vi "Terminate Sequence.vi"(4 "Buffers":T1, 6 "Terminal Options":T2={"Implied CR with LF"=TRUE, "Local Echo"=FALSE, "Tab Width"=8, "Color Scheme"={"Black"=2302755, "Red"=16711695, "Green"=9232651, "Yellow"=16759040, "Blue"=36344, "Magenta"=7160742, "Cyan"=55531, "White"=15132390, "Bright Black"=4473924, "Bright Red"=16721728, "Bright Green"=11264347, "Bright Yellow"=16765506, "Bright Blue"=37631, "Bright Magenta"=10117099, "Bright Cyan"=6815728, "Bright White"=16777215}, "Default FG"=37, "Default BG"=90, "History Length"=5000, "Font Face"="Fixedsys", "Font Size"=14, "Rows"=24, "Cols"=80} {"Default BG" items=["Black"=30, "Red"=31, "Green"=32, "Yellow"=33, "Blue"=34, "Magenta"=35, "Cyan"=36, "White"=37, "Gray"=90, "Bright Red"=91, "Bright Green"=92, "Bright Yellow"=93, "Bright Blue"=94, "Bright Magenta"=95, "Bright Cyan"=96, "Bright White"=97]; "Default FG" items=["Black"=30, "Red"=31, "Green"=32, "Yellow"=33, "Blue"=34, "Magenta"=35, "Cyan"=36, "White"=37, "Gray"=90, "Bright Red"=91, "Bright Green"=92, "Bright Yellow"=93, "Bright Blue"=94, "Bright Magenta"=95, "Bright Cyan"=96, "Bright White"=97]}, 10 "Terminator":u8, 11 "Parse State In":T5) -> (3 "Parse State":T5)   [LabVIEW 2020, in "Terminal.lvlib" / "Terminal.lvclass"]
uses:
  Terminal.lvclass
  Terminal.lvclass/Terminal.ctl
  Color.ctl
  Terminal.lvlib
  TermBuffer/TermBuffer.lvclass
  Buffer.ctl
  Parse State.ctl
  Color Scheme.ctl
  Terminal Options.ctl
  Buffers.ctl
  Position.ctl
  Cursor.ctl
  Text Attributes.ctl
  Buffer State.ctl
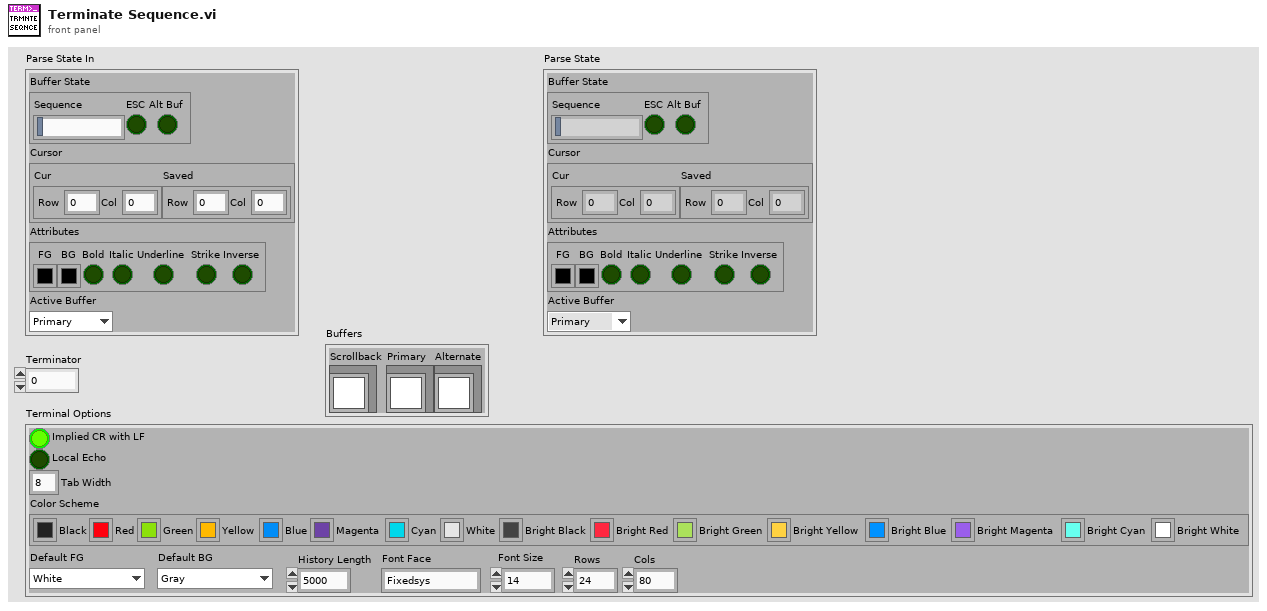
[diagram p1: front panel]
types:
  T1 = typedef "Terminal.lvlib/Terminal.lvclass/Buffers.ctl" = cluster{"Scrollback":refnum<class "TermBuffer.lvclass">, "Primary":refnum<class "TermBuffer.lvclass">, "Alternate":refnum<class "TermBuffer.lvclass">}
  T2 = typedef "Terminal.lvlib/Terminal Options.ctl" = cluster{"Implied CR with LF":bool, "Local Echo":bool, "Tab Width":i32, "Color Scheme":T3, "Default FG":T4, "Default BG":T4, "History Length":i32, "Font Face":string, "Font Size":i16, "Rows":i32, "Cols":i32}
  T3 = typedef "Terminal.lvlib/Color Scheme.ctl" = cluster{"Black":u32, "Red":u32, "Green":u32, "Yellow":u32, "Blue":u32, "Magenta":u32, "Cyan":u32, "White":u32, "Bright Black":u32, "Bright Red":u32, "Bright Green":u32, "Bright Yellow":u32, "Bright Blue":u32, "Bright Magenta":u32, "Bright Cyan":u32, "Bright White":u32}
  T4 = typedef "Terminal.lvlib/Color.ctl" = i8
  T5 = typedef "Terminal.lvlib/Terminal.lvclass/Parse State.ctl" = cluster{"Buffer State":T6, "Cursor":T7, "Attributes":T9, "Active Buffer":T10}
  T6 = typedef "Terminal.lvlib/Terminal.lvclass/Buffer State.ctl" = cluster{"Sequence":string, "ESC":bool, "Alt Buf":bool}
  T7 = typedef "Terminal.lvlib/Terminal.lvclass/Cursor.ctl" = cluster{"Cur":T8, "Saved":T8}
  T8 = typedef "Terminal.lvlib/Terminal.lvclass/Position.ctl" = cluster{"Row":i32, "Col":i32}
  T9 = typedef "Terminal.lvlib/Text Attributes.ctl" = cluster{"FG":u32, "BG":u32, "Bold":bool, "Italic":bool, "Underline":bool, "Strike":bool, "Inverse":bool}
  T10 = typedef "Terminal.lvlib/Buffer.ctl" = enum16{"Primary", "Alternate"}
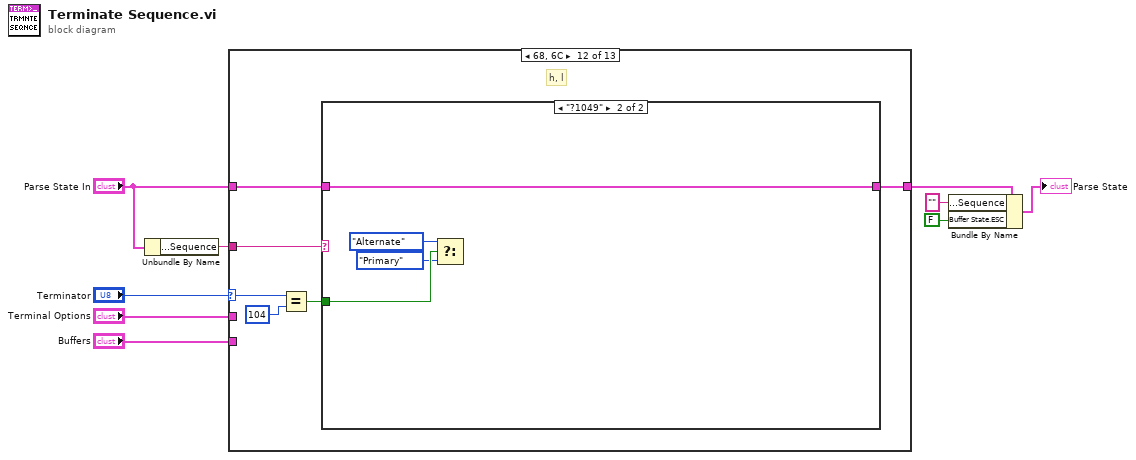
[diagram p0: block diagram]
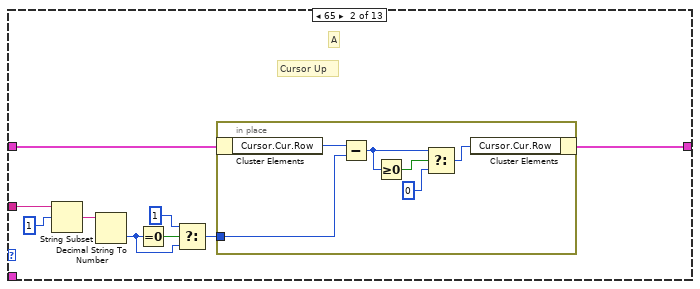
[diagram p3: hidden frame]
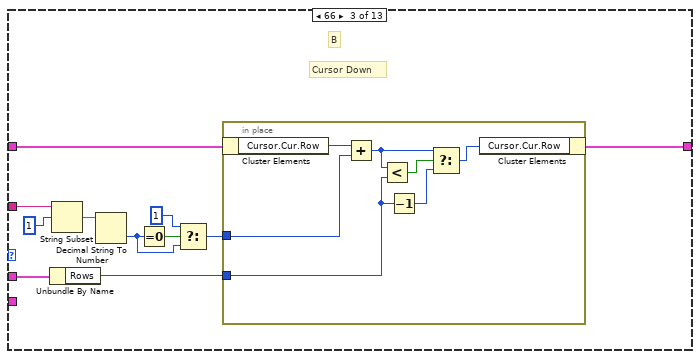
[diagram p4: hidden frame]
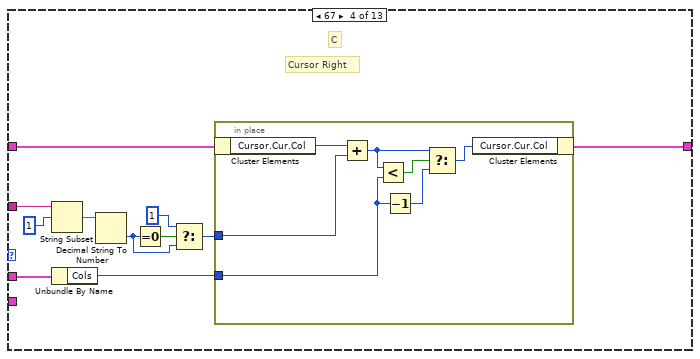
[diagram p5: hidden frame]
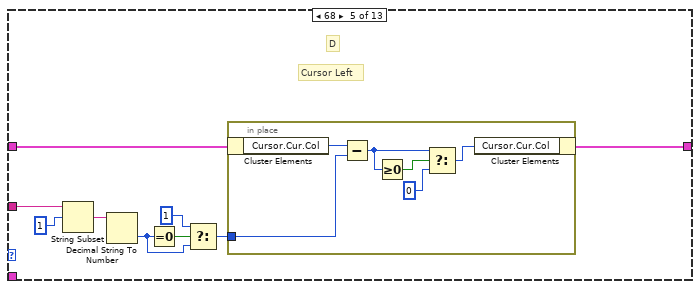
[diagram p6: hidden frame]
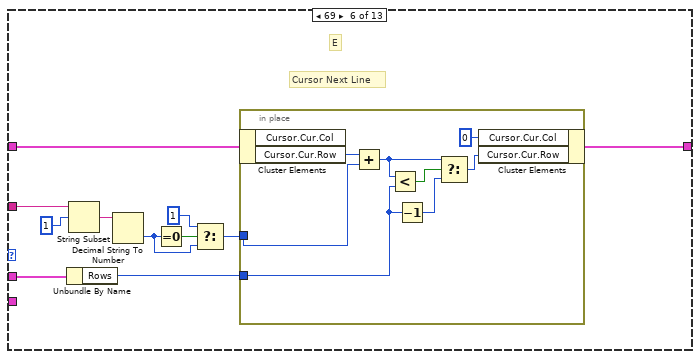
[diagram p7: hidden frame]
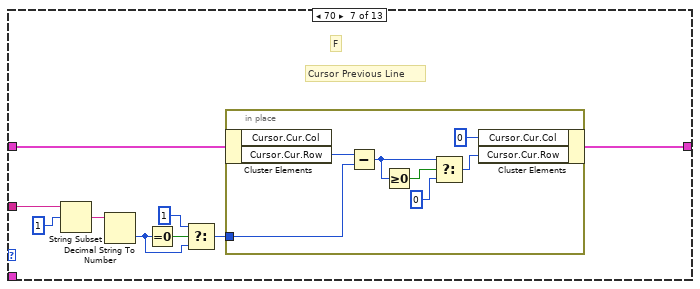
[diagram p8: hidden frame]
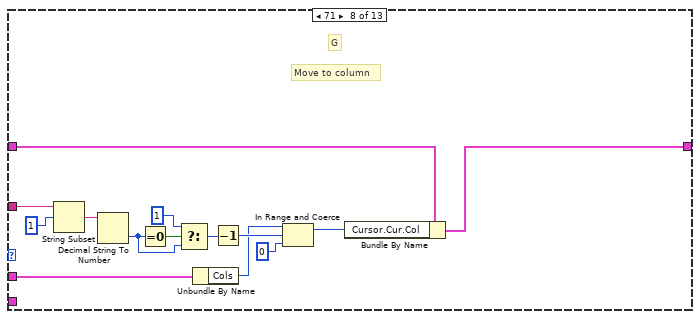
[diagram p9: hidden frame]
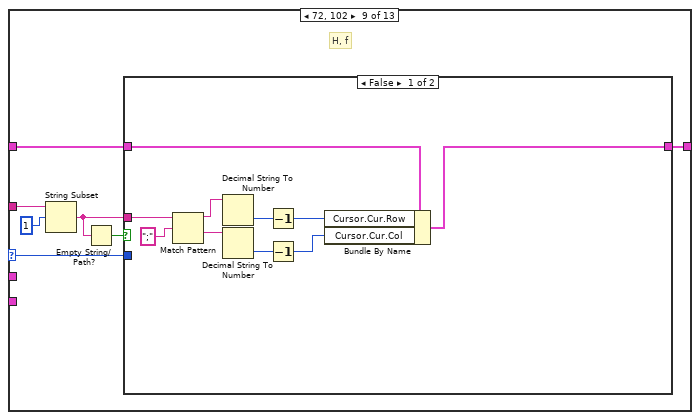
[diagram p10: hidden frame]
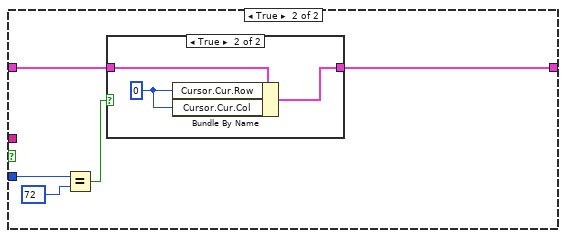
[diagram p11: hidden frame]
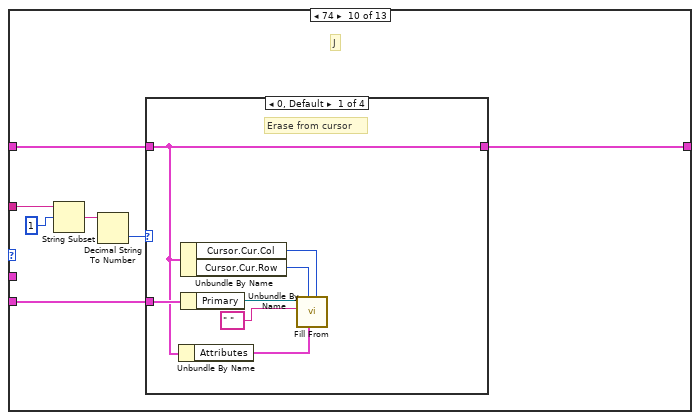
[diagram p13: hidden frame]
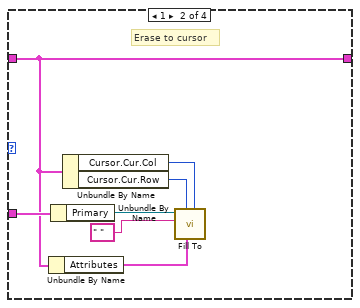
[diagram p14: hidden frame]
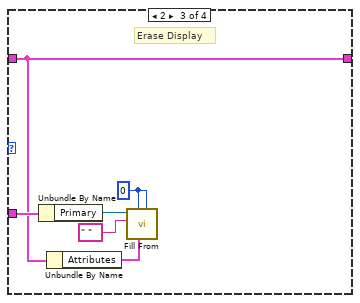
[diagram p15: hidden frame]
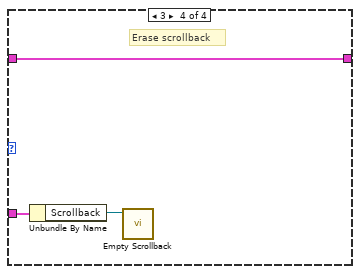
[diagram p16: hidden frame]
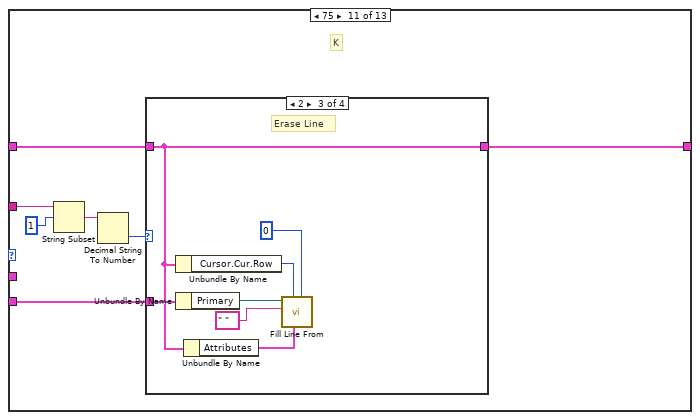
[diagram p17: hidden frame]
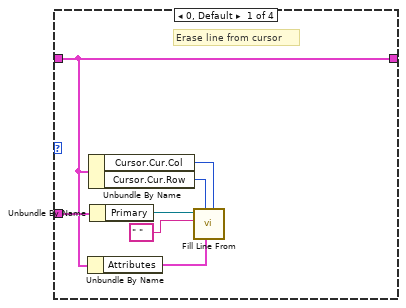
[diagram p18: hidden frame]
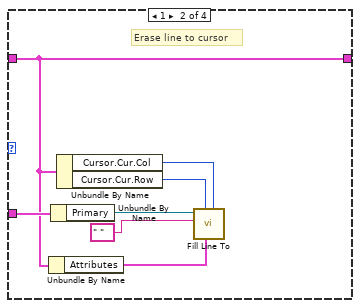
[diagram p19: hidden frame]
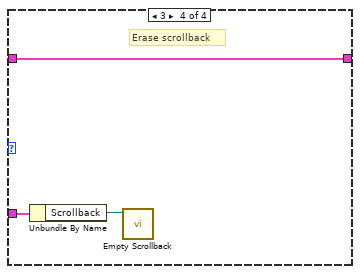
[diagram p20: hidden frame]
diagram:
  n1 = Unbundle By Name("Parse State In") -> ("Buffer State.Sequence"=w7:string)
  n2 = case shown="68, 6C" "Terminator" {
    selector: "Terminator" -> [_ _ _ _ _ _ _ _ w126 _ _ w216 _]
    tunnel: "Parse State In" -> [w10 w16 w33 w51 w63 w80 w97 w114 w130 w155 w185 w218 w226]
    tunnel: w7 -> [_ w19 w36 w54 w64 w79 w98 w120 w132 w156 w186 w214 w229]
    tunnel: [w10 w15 w32 w50 w62 w77 w96 w112 w128 w152 w182 w217 w225] -> w6
    tunnel: "Terminal Options" -> [_ _ w31 w49 _ w78 _ w116 _ _ _ _ w224]
    tunnel: "Buffers" -> [_ _ _ _ _ _ _ _ _ w153 w183 _ _]
    frame Default {
    }
    frame 65 {
      # "Cursor Up"
      # "A"
      n3 = String Subset(string=w19, offset (0)=1) -> (substring=w17:string)  [unwired: 1 in]
      n4 = Decimal String To Number(string=w17) -> (number=w12:i32)  [unwired: 2 in, 1 out]
      n5 = Equal To 0?(x=w12) -> (x = 0?=w14:bool)
      n6 = Select(t=1, s=w14, f=w12) -> (s? t:f=w11:i32)
      n7 = in-place {
        in-place-border: w11 -> [w24]
        n8 = in-place-cluster #1(w16) -> ("Cursor.Cur.Row"=w25:i32)
        n9 = Subtract(x=w25, y=w24) -> (x-y=w22:i32)
        n10 = Greater Or Equal To 0?(x=w22) -> (x >= 0?=w23:bool)
        n11 = Select(t=w22, s=w23, f=0) -> (s? t:f=w20:i32)
        n12 = in-place-cluster #1("Cursor.Cur.Row"=w20) -> (w15:T5)
      }
    }
    frame 66 {
      # "Cursor Down"
      # "B"
      n13 = Unbundle By Name(w31) -> ("Rows"=w30:i32)
      n14 = String Subset(string=w36, offset (0)=1) -> (substring=w34:string)  [unwired: 1 in]
      n15 = Decimal String To Number(string=w34) -> (number=w27:i32)  [unwired: 2 in, 1 out]
      n16 = Equal To 0?(x=w27) -> (x = 0?=w29:bool)
      n17 = Select(t=1, s=w29, f=w27) -> (s? t:f=w26:i32)
      n18 = in-place {
        in-place-border: w30 -> [w39]
        in-place-border: w26 -> [w37]
        n19 = in-place-cluster #2(w33) -> ("Cursor.Cur.Row"=w43:i32)
        n20 = Add(x=w43, y=w37) -> (x+y=w41:i32)
        n21 = Less?(x=w41, y=w39) -> (x < y?=w40:bool)
        n22 = Decrement(x=w39) -> (x-1=w38:i32)
        n23 = Select(t=w41, s=w40, f=w38) -> (s? t:f=w42:i32)
        n24 = in-place-cluster #2("Cursor.Cur.Row"=w42) -> (w32:T5)
      }
    }
    frame 67 {
      # "Cursor Right"
      # "C"
      n25 = String Subset(string=w54, offset (0)=1) -> (substring=w52:string)  [unwired: 1 in]
      n26 = Unbundle By Name(w49) -> ("Cols"=w48:i32)
      n27 = Decimal String To Number(string=w52) -> (number=w46:i32)  [unwired: 2 in, 1 out]
      n28 = Equal To 0?(x=w46) -> (x = 0?=w47:bool)
      n29 = Select(t=1, s=w47, f=w46) -> (s? t:f=w44:i32)
      n30 = in-place {
        in-place-border: w44 -> [w60]
        in-place-border: w48 -> [w56]
        n31 = in-place-cluster #3(w51) -> ("Cursor.Cur.Col"=w61:i32)
        n32 = Add(x=w61, y=w60) -> (x+y=w58:i32)
        n33 = Less?(x=w58, y=w56) -> (x < y?=w57:bool)
        n34 = Decrement(x=w56) -> (x-1=w55:i32)
        n35 = Select(t=w58, s=w57, f=w55) -> (s? t:f=w59:i32)
        n36 = in-place-cluster #3("Cursor.Cur.Col"=w59) -> (w50:T5)
      }
    }
    frame 68 {
      # "Cursor Left"
      # "D"
      n37 = String Subset(string=w64, offset (0)=1) -> (substring=w69:string)  [unwired: 1 in]
      n38 = Decimal String To Number(string=w69) -> (number=w66:i32)  [unwired: 2 in, 1 out]
      n39 = Equal To 0?(x=w66) -> (x = 0?=w68:bool)
      n40 = Select(t=1, s=w68, f=w66) -> (s? t:f=w65:i32)
      n41 = in-place {
        in-place-border: w65 -> [w75]
        n42 = in-place-cluster #4(w63) -> ("Cursor.Cur.Col"=w76:i32)
        n43 = Subtract(x=w76, y=w75) -> (x-y=w73:i32)
        n44 = Greater Or Equal To 0?(x=w73) -> (x >= 0?=w74:bool)
        n45 = Select(t=w73, s=w74, f=0) -> (s? t:f=w71:i32)
        n46 = in-place-cluster #4("Cursor.Cur.Col"=w71) -> (w62:T5)
      }
    }
    frame 69 {
      # "Cursor Next Line"
      # "E"
      n47 = Unbundle By Name(w78) -> ("Rows"=w85:i32)
      n48 = String Subset(string=w79, offset (0)=1) -> (substring=w86:string)  [unwired: 1 in]
      n49 = Decimal String To Number(string=w86) -> (number=w82:i32)  [unwired: 2 in, 1 out]
      n50 = Equal To 0?(x=w82) -> (x = 0?=w84:bool)
      n51 = Select(t=1, s=w84, f=w82) -> (s? t:f=w81:i32)
      n52 = in-place {
        in-place-border: w85 -> [w91]
        in-place-border: w81 -> [w89]
        n53 = in-place-cluster #5(w80) -> ("Cursor.Cur.Row"=w95:i32)  [unwired: 1 out]
        n54 = Add(x=w95, y=w89) -> (x+y=w93:i32)
        n55 = Less?(x=w93, y=w91) -> (x < y?=w92:bool)
        n56 = Decrement(x=w91) -> (x-1=w90:i32)
        n57 = Select(t=w93, s=w92, f=w90) -> (s? t:f=w94:i32)
        n58 = in-place-cluster #5("Cursor.Cur.Col"=0 ("Cur Col"), "Cursor.Cur.Row"=w94) -> (w77:T5)
      }
    }
    frame 70 {
      # "Cursor Previous Line"
      # "F"
      n59 = String Subset(string=w98, offset (0)=1) -> (substring=w103:string)  [unwired: 1 in]
      n60 = Decimal String To Number(string=w103) -> (number=w100:i32)  [unwired: 2 in, 1 out]
      n61 = Equal To 0?(x=w100) -> (x = 0?=w102:bool)
      n62 = Select(t=1, s=w102, f=w100) -> (s? t:f=w99:i32)
      n63 = in-place {
        in-place-border: w99 -> [w110]
        n64 = in-place-cluster #6(w97) -> ("Cursor.Cur.Row"=w111:i32)  [unwired: 1 out]
        n65 = Subtract(x=w111, y=w110) -> (x-y=w108:i32)
        n66 = Greater Or Equal To 0?(x=w108) -> (x >= 0?=w109:bool)
        n67 = Select(t=w108, s=w109, f=0) -> (s? t:f=w106:i32)
        n68 = in-place-cluster #6("Cursor.Cur.Col"=0 ("Cur Col"), "Cursor.Cur.Row"=w106) -> (w96:T5)
      }
    }
    frame 71 {
      # "Move to column"
      # "G"
      n69 = String Subset(string=w120, offset (0)=1) -> (substring=w124:string)  [unwired: 1 in]
      n70 = Decimal String To Number(string=w124) -> (number=w121:i32)  [unwired: 2 in, 1 out]
      n71 = Equal To 0?(x=w121) -> (x = 0?=w123:bool)
      n72 = Select(t=1, s=w123, f=w121) -> (s? t:f=w119:i32)
      n73 = Unbundle By Name(w116) -> ("Cols"=w115:i32)
      n74 = Decrement(x=w119) -> (x-1=w118:i32)
      n75 = In Range and Coerce(upper limit=w115, x=w118, lower limit=0) -> (coerced(x)=w113:i32)  [unwired: 1 out]
      n76 = Bundle By Name(cluster=w114, "Cursor.Cur.Col"=w113) -> (w112:T5)
    }
    frame 72, 102 {
      # "H, f"
      n77 = String Subset(string=w132, offset (0)=1) -> (substring=w127:string)  [unwired: 1 in]
      n78 = Empty String/Path?(string/path=w127) -> (empty?=w129:bool)
      n79 = case shown="False" w129 {
        tunnel: w130 -> [w138 w147]
        tunnel: [w135 w146] -> w128
        tunnel: w127 -> [w142 _]
        tunnel: w126 -> [_ w145]
        frame False {
          n80 = Match Pattern(string=w142, regular expression=";") -> (before substring=w139:string, after substring=w140:string)  [unwired: 1 in, 2 out]
          n81 = Decimal String To Number(string=w139) -> (number=w137:i32)  [unwired: 2 in, 1 out]
          n82 = Decimal String To Number(string=w140) -> (number=w136:i32)  [unwired: 2 in, 1 out]
          n83 = Decrement(x=w137) -> (x-1=w134:i32)
          n84 = Decrement(x=w136) -> (x-1=w133:i32)
          n85 = Bundle By Name(cluster=w138, "Cursor.Cur.Row"=w134, "Cursor.Cur.Col"=w133) -> (w135:T5)
        }
        frame True {
          n86 = Equal?(x=w145, y=u8 72) -> (x = y?=w143:bool)
          n87 = case shown="True" w143 {
            tunnel: w147 -> [w148 w151]
            tunnel: [w148 w149] -> w146
            frame False {
            }
            frame True {
              w150 = 0 ("Cur Row")
              n88 = Bundle By Name(cluster=w151, "Cursor.Cur.Row"=w150, "Cursor.Cur.Col"=w150) -> (w149:T5)
            }
          }
        }
      }
    }
    frame 74 {
      # "J"
      n89 = String Subset(string=w156, offset (0)=1) -> (substring=w157:string)  [unwired: 1 in]
      n90 = Decimal String To Number(string=w157) -> (number=w154:i32)  [unwired: 2 in, 1 out]
      n91 = case shown="0, Default" w154 {
        tunnel: w155 -> [w161 w166 w174 w181]
        tunnel: w153 -> [w165 w167 w178 w180]
        tunnel: [w161 w166 w174 w181] -> w152
        frame 0, Default {
          # "Erase from cursor"
          n92 = Unbundle By Name(w161) -> ("Attributes"=w159:T9)
          n93 = Unbundle By Name(w161) -> ("Cursor.Cur.Col"=w162:i32, "Cursor.Cur.Row"=w163:i32)
          n94 = Unbundle By Name(w165) -> ("Primary"=w164:refnum<class "TermBuffer.lvclass">)
          n95 = call "Fill From.vi"("Col"=w162, "Attributes"=w159, "Row"=w163, "Char"=" ", "TermBuffer in"=w164) -> ()  [unwired: 5 in, 2 out]
        }
        frame 1 {
          # "Erase to cursor"
          n96 = Unbundle By Name(w166) -> ("Attributes"=w168:T9)
          n97 = Unbundle By Name(w167) -> ("Primary"=w172:refnum<class "TermBuffer.lvclass">)
          n98 = Unbundle By Name(w166) -> ("Cursor.Cur.Col"=w170:i32, "Cursor.Cur.Row"=w171:i32)
          n99 = call "Fill To.vi"("Col"=w170, "Attributes"=w168, "Row"=w171, "Char"=" ", "TermBuffer in"=w172) -> ()  [unwired: 5 in, 2 out]
        }
        frame 2 {
          w175 = 0 ("Row")
          # "Erase Display"
          n100 = Unbundle By Name(w178) -> ("Primary"=w177:refnum<class "TermBuffer.lvclass">)
          n101 = Unbundle By Name(w174) -> ("Attributes"=w173:T9)
          n102 = call "Fill From.vi"("Col"=w175, "Attributes"=w173, "Row"=w175, "Char"=" ", "TermBuffer in"=w177) -> ()  [unwired: 5 in, 2 out]
        }
        frame 3 {
          # "Erase scrollback"
          n103 = Unbundle By Name(w180) -> ("Scrollback"=w179:refnum<class "TermBuffer.lvclass">)
          n104 = call "Empty Scrollback.vi"("TermBuffer in"=w179) -> ()  [unwired: 9 in, 2 out]
        }
      }
    }
    frame 75 {
      # "K"
      n105 = String Subset(string=w186, offset (0)=1) -> (substring=w187:string)  [unwired: 1 in]
      n106 = Decimal String To Number(string=w187) -> (number=w184:i32)  [unwired: 2 in, 1 out]
      n107 = case shown="2" w184 {
        tunnel: w185 -> [w191 w196 w206 w212]
        tunnel: w183 -> [w195 w197 w209 w211]
        tunnel: [w191 w196 w206 w212] -> w182
        frame 0, Default {
          # "Erase line from cursor"
          n108 = Unbundle By Name(w191) -> ("Attributes"=w189:T9)
          n109 = Unbundle By Name(w191) -> ("Cursor.Cur.Col"=w192:i32, "Cursor.Cur.Row"=w193:i32)
          n110 = Unbundle By Name(w195) -> ("Primary"=w194:refnum<class "TermBuffer.lvclass">)
          n111 = call "Fill Line From.vi"("Col"=w192, "Attributes"=w189, "Row"=w193, "Char"=" ", "TermBuffer in"=w194) -> ()  [unwired: 5 in, 2 out]
        }
        frame 1 {
          # "Erase line to cursor"
          n112 = Unbundle By Name(w196) -> ("Attributes"=w198:T9)
          n113 = Unbundle By Name(w197) -> ("Primary"=w202:refnum<class "TermBuffer.lvclass">)
          n114 = Unbundle By Name(w196) -> ("Cursor.Cur.Col"=w200:i32, "Cursor.Cur.Row"=w201:i32)
          n115 = call "Fill Line To.vi"("Col"=w200, "Attributes"=w198, "Row"=w201, "Char"=" ", "TermBuffer in"=w202) -> ()  [unwired: 5 in, 2 out]
        }
        frame 2 {
          # "Erase Line"
          n116 = Unbundle By Name(w206) -> ("Cursor.Cur.Row"=w205:i32)
          n117 = Unbundle By Name(w209) -> ("Primary"=w208:refnum<class "TermBuffer.lvclass">)
          n118 = Unbundle By Name(w206) -> ("Attributes"=w203:T9)
          n119 = call "Fill Line From.vi"("Col"=0, "Attributes"=w203, "Row"=w205, "Char"=" ", "TermBuffer in"=w208) -> ()  [unwired: 5 in, 2 out]
        }
        frame 3 {
          # "Erase scrollback"
          n120 = Unbundle By Name(w211) -> ("Scrollback"=w210:refnum<class "TermBuffer.lvclass">)
          n121 = call "Empty Scrollback.vi"("TermBuffer in"=w210) -> ()  [unwired: 9 in, 2 out]
        }
      }
    }
    frame 104, 108 {
      # "h, l"
      n122 = Equal?(x=w216, y=u8 104) -> (x = y?=w213:bool)
      n123 = case shown="\"?1049\"" w214 {
        tunnel: w218 -> [w219 w220]
        tunnel: [w219 w220] -> w217
        tunnel: w213 -> [_ w223]
        frame Default {
        }
        frame "?1049" {
          n124 = Select(t=Buffer."Alternate" ("Buffer"), s=w223, f=Buffer."Primary" ("Buffer")) -> ()  [unwired: 1 out]
        }
      }
    }
    frame 109 {
      w230 = 1 ("length (rest)")
      # "Character mode / color"
      # "m"
      n125 = String Subset(string=w229, offset (0)=w230) -> (substring=w228:string)  [unwired: 1 in]
      n126 = String Subset(string=w229, length (rest)=w230) -> (substring=w232:string)  [unwired: 1 in]
      n127 = Equal?(x=w232, y="[") -> (x = y?=w227:bool)
      n128 = case shown="True" w227 {
        tunnel: w228 -> [_ w239]
        tunnel: w226 -> [w233 w236]
        tunnel: [w233 w235] -> w225
        tunnel: w224 -> [_ w234]
        frame False {
        }
        frame True {
          n129 = call <vilib>:"Delimited String to 1D String Array.vi"("delimiter"=";", "delimited string"=w239) -> ("string array"=w237:string[])  [unwired: 9 in]
          n130 = for {
            tunnel: w237 -> [w242] mode=indexing
            shift-right: [w241] -> w235
            shift-left: w236 -> [w243]
            tunnel: w234 -> [w240]
            n131 = case shown="\"0\"" w242 {
              tunnel: w243 -> [w244 w253 w256 w257 w260 w263 w264 w267 w268 w271 w274 w277 w280 w281 w284 w285 w288 w291 w297 w303 w309 w315 w321 w327 w333 w340 w345 w351 w357 w363 w369 w375 w381 w387 w394 w399 w405 w411 w417 w423 w429 w435 w441 w447 w453 w459 w465 w471 w477 w483 w489]
              tunnel: [w244 w251 w254 w257 w258 w261 w264 w265 w268 w269 w272 w276 w278 w281 w282 w285 w286 w289 w295 w301 w307 w313 w319 w325 w331 w338 w343 w349 w355 w361 w367 w373 w379 w385 w392 w397 w403 w409 w415 w421 w427 w433 w439 w445 w451 w457 w463 w469 w475 w481 w487] -> w241
              tunnel: w240 -> [_ w250 _ _ _ _ _ _ _ _ _ _ _ _ _ _ _ w294 w300 w306 w312 w318 w324 w330 w336 w342 w348 w354 w360 w366 w372 w378 w384 w390 w396 w402 w408 w414 w420 w426 w432 w438 w444 w450 w456 w462 w468 w474 w480 w486 w492]
              frame Default {
              }
              frame "0" {
                w252 = FALSE ("Bold")
                n132 = Unbundle By Name(w250) -> ("Color Scheme"=w247:T3, "Default FG"=w249:T4, "Default BG"=w248:T4)
                n133 = call "Select Color.vi"("Color"=w249, "Color Scheme"=w247) -> ("Color Value"=w246:u32)  [unwired: 9 in]
                n134 = call "Select Color.vi"("Color"=w248, "Color Scheme"=w247) -> ("Color Value"=w245:u32)  [unwired: 9 in]
                n135 = Bundle By Name(cluster=w253, "Attributes.Bold"=w252, "Attributes.Italic"=w252, "Attributes.Underline"=w252, "Attributes.Strike"=w252, "Attributes.Inverse"=w252, "Attributes.FG"=w246, "Attributes.BG"=w245) -> (w251:T5)
              }
              frame "1" {
                n136 = Bundle By Name(cluster=w256, "Attributes.Bold"=TRUE ("Bold")) -> (w254:T5)
              }
              frame "2" {
                # "Dim/Faint On"
              }
              frame "3" {
                n137 = Bundle By Name(cluster=w260, "Attributes.Italic"=TRUE ("Italic")) -> (w258:T5)
              }
              frame "4" {
                n138 = Bundle By Name(cluster=w263, "Attributes.Underline"=TRUE ("Underline")) -> (w261:T5)
              }
              frame "5" {
                # "#TODO\nBlink On"
              }
              frame "7" {
                n139 = Bundle By Name(cluster=w267, "Attributes.Inverse"=TRUE ("Inverse")) -> (w265:T5)
              }
              frame "8" {
                # "Invisible On"
              }
              frame "9" {
                n140 = Bundle By Name(cluster=w271, "Attributes.Strike"=TRUE ("Strike")) -> (w269:T5)
              }
              frame "22" {
                n141 = Bundle By Name(cluster=w274, "Attributes.Bold"=FALSE ("Bold")) -> (w272:T5)
              }
              frame "23" {
                n142 = Bundle By Name(cluster=w277, "Attributes.Italic"=FALSE ("Italic")) -> (w276:T5)
              }
              frame "24" {
                n143 = Bundle By Name(cluster=w280, "Attributes.Underline"=FALSE ("Underline")) -> (w278:T5)
              }
              frame "25" {
                # "#TODO\nBlink Off"
              }
              frame "27" {
                n144 = Bundle By Name(cluster=w284, "Attributes.Inverse"=FALSE ("Inverse")) -> (w282:T5)
              }
              frame "28" {
                # "Invisible Off"
              }
              frame "29" {
                n145 = Bundle By Name(cluster=w288, "Attributes.Strike"=FALSE ("Strike")) -> (w286:T5)
              }
              frame "30" {
                w292 = T4 30 items=["Black"=30, "Red"=31, "Green"=32, "Yellow"=33, "Blue"=34, "Magenta"=35, "Cyan"=36, "White"=37, "Gray"=90, "Bright Red"=91, "Bright Green"=92, "Bright Yellow"=93, "Bright Blue"=94, "Bright Magenta"=95, "Bright Cyan"=96, "Bright White"=97] ("Color")
                n146 = Unbundle By Name(w294) -> ("Color Scheme"=w293:T3)
                n147 = call "Select Color.vi"("Color"=w292, "Color Scheme"=w293) -> ("Color Value"=w290:u32)  [unwired: 9 in]
                n148 = Bundle By Name(cluster=w291, "Attributes.FG"=w290) -> (w289:T5)
              }
              frame "31" {
                w298 = T4 31 items=["Black"=30, "Red"=31, "Green"=32, "Yellow"=33, "Blue"=34, "Magenta"=35, "Cyan"=36, "White"=37, "Gray"=90, "Bright Red"=91, "Bright Green"=92, "Bright Yellow"=93, "Bright Blue"=94, "Bright Magenta"=95, "Bright Cyan"=96, "Bright White"=97] ("Color")
                n149 = Unbundle By Name(w300) -> ("Color Scheme"=w299:T3)
                n150 = call "Select Color.vi"("Color"=w298, "Color Scheme"=w299) -> ("Color Value"=w296:u32)  [unwired: 9 in]
                n151 = Bundle By Name(cluster=w297, "Attributes.FG"=w296) -> (w295:T5)
              }
              frame "32" {
                w304 = T4 32 items=["Black"=30, "Red"=31, "Green"=32, "Yellow"=33, "Blue"=34, "Magenta"=35, "Cyan"=36, "White"=37, "Gray"=90, "Bright Red"=91, "Bright Green"=92, "Bright Yellow"=93, "Bright Blue"=94, "Bright Magenta"=95, "Bright Cyan"=96, "Bright White"=97] ("Color")
                n152 = Unbundle By Name(w306) -> ("Color Scheme"=w305:T3)
                n153 = call "Select Color.vi"("Color"=w304, "Color Scheme"=w305) -> ("Color Value"=w302:u32)  [unwired: 9 in]
                n154 = Bundle By Name(cluster=w303, "Attributes.FG"=w302) -> (w301:T5)
              }
              frame "33" {
                w310 = T4 33 items=["Black"=30, "Red"=31, "Green"=32, "Yellow"=33, "Blue"=34, "Magenta"=35, "Cyan"=36, "White"=37, "Gray"=90, "Bright Red"=91, "Bright Green"=92, "Bright Yellow"=93, "Bright Blue"=94, "Bright Magenta"=95, "Bright Cyan"=96, "Bright White"=97] ("Color")
                n155 = Unbundle By Name(w312) -> ("Color Scheme"=w311:T3)
                n156 = call "Select Color.vi"("Color"=w310, "Color Scheme"=w311) -> ("Color Value"=w308:u32)  [unwired: 9 in]
                n157 = Bundle By Name(cluster=w309, "Attributes.FG"=w308) -> (w307:T5)
              }
              frame "34" {
                w316 = T4 34 items=["Black"=30, "Red"=31, "Green"=32, "Yellow"=33, "Blue"=34, "Magenta"=35, "Cyan"=36, "White"=37, "Gray"=90, "Bright Red"=91, "Bright Green"=92, "Bright Yellow"=93, "Bright Blue"=94, "Bright Magenta"=95, "Bright Cyan"=96, "Bright White"=97] ("Color")
                n158 = Unbundle By Name(w318) -> ("Color Scheme"=w317:T3)
                n159 = call "Select Color.vi"("Color"=w316, "Color Scheme"=w317) -> ("Color Value"=w314:u32)  [unwired: 9 in]
                n160 = Bundle By Name(cluster=w315, "Attributes.FG"=w314) -> (w313:T5)
              }
              frame "35" {
                w322 = T4 35 items=["Black"=30, "Red"=31, "Green"=32, "Yellow"=33, "Blue"=34, "Magenta"=35, "Cyan"=36, "White"=37, "Gray"=90, "Bright Red"=91, "Bright Green"=92, "Bright Yellow"=93, "Bright Blue"=94, "Bright Magenta"=95, "Bright Cyan"=96, "Bright White"=97] ("Color")
                n161 = Unbundle By Name(w324) -> ("Color Scheme"=w323:T3)
                n162 = call "Select Color.vi"("Color"=w322, "Color Scheme"=w323) -> ("Color Value"=w320:u32)  [unwired: 9 in]
                n163 = Bundle By Name(cluster=w321, "Attributes.FG"=w320) -> (w319:T5)
              }
              frame "36" {
                w328 = T4 36 items=["Black"=30, "Red"=31, "Green"=32, "Yellow"=33, "Blue"=34, "Magenta"=35, "Cyan"=36, "White"=37, "Gray"=90, "Bright Red"=91, "Bright Green"=92, "Bright Yellow"=93, "Bright Blue"=94, "Bright Magenta"=95, "Bright Cyan"=96, "Bright White"=97] ("Color")
                n164 = Unbundle By Name(w330) -> ("Color Scheme"=w329:T3)
                n165 = call "Select Color.vi"("Color"=w328, "Color Scheme"=w329) -> ("Color Value"=w326:u32)  [unwired: 9 in]
                n166 = Bundle By Name(cluster=w327, "Attributes.FG"=w326) -> (w325:T5)
              }
              frame "37" {
                w334 = T4 37 items=["Black"=30, "Red"=31, "Green"=32, "Yellow"=33, "Blue"=34, "Magenta"=35, "Cyan"=36, "White"=37, "Gray"=90, "Bright Red"=91, "Bright Green"=92, "Bright Yellow"=93, "Bright Blue"=94, "Bright Magenta"=95, "Bright Cyan"=96, "Bright White"=97] ("Color")
                n167 = Unbundle By Name(w336) -> ("Color Scheme"=w335:T3)
                n168 = call "Select Color.vi"("Color"=w334, "Color Scheme"=w335) -> ("Color Value"=w332:u32)  [unwired: 9 in]
                n169 = Bundle By Name(cluster=w333, "Attributes.FG"=w332) -> (w331:T5)
              }
              frame "39" {
                n170 = Unbundle By Name(w342) -> ("Color Scheme"=w341:T3, "Default FG"=w337:T4)
                n171 = call "Select Color.vi"("Color"=w337, "Color Scheme"=w341) -> ("Color Value"=w339:u32)  [unwired: 9 in]
                n172 = Bundle By Name(cluster=w340, "Attributes.FG"=w339) -> (w338:T5)
              }
              frame "40" {
                w346 = T4 30 items=["Black"=30, "Red"=31, "Green"=32, "Yellow"=33, "Blue"=34, "Magenta"=35, "Cyan"=36, "White"=37, "Gray"=90, "Bright Red"=91, "Bright Green"=92, "Bright Yellow"=93, "Bright Blue"=94, "Bright Magenta"=95, "Bright Cyan"=96, "Bright White"=97] ("Color")
                n173 = Unbundle By Name(w348) -> ("Color Scheme"=w347:T3)
                n174 = call "Select Color.vi"("Color"=w346, "Color Scheme"=w347) -> ("Color Value"=w344:u32)  [unwired: 9 in]
                n175 = Bundle By Name(cluster=w345, "Attributes.BG"=w344) -> (w343:T5)
              }
              frame "41" {
                w352 = T4 31 items=["Black"=30, "Red"=31, "Green"=32, "Yellow"=33, "Blue"=34, "Magenta"=35, "Cyan"=36, "White"=37, "Gray"=90, "Bright Red"=91, "Bright Green"=92, "Bright Yellow"=93, "Bright Blue"=94, "Bright Magenta"=95, "Bright Cyan"=96, "Bright White"=97] ("Color")
                n176 = Unbundle By Name(w354) -> ("Color Scheme"=w353:T3)
                n177 = call "Select Color.vi"("Color"=w352, "Color Scheme"=w353) -> ("Color Value"=w350:u32)  [unwired: 9 in]
                n178 = Bundle By Name(cluster=w351, "Attributes.BG"=w350) -> (w349:T5)
              }
              frame "42" {
                w358 = T4 32 items=["Black"=30, "Red"=31, "Green"=32, "Yellow"=33, "Blue"=34, "Magenta"=35, "Cyan"=36, "White"=37, "Gray"=90, "Bright Red"=91, "Bright Green"=92, "Bright Yellow"=93, "Bright Blue"=94, "Bright Magenta"=95, "Bright Cyan"=96, "Bright White"=97] ("Color")
                n179 = Unbundle By Name(w360) -> ("Color Scheme"=w359:T3)
                n180 = call "Select Color.vi"("Color"=w358, "Color Scheme"=w359) -> ("Color Value"=w356:u32)  [unwired: 9 in]
                n181 = Bundle By Name(cluster=w357, "Attributes.BG"=w356) -> (w355:T5)
              }
              frame "43" {
                w364 = T4 33 items=["Black"=30, "Red"=31, "Green"=32, "Yellow"=33, "Blue"=34, "Magenta"=35, "Cyan"=36, "White"=37, "Gray"=90, "Bright Red"=91, "Bright Green"=92, "Bright Yellow"=93, "Bright Blue"=94, "Bright Magenta"=95, "Bright Cyan"=96, "Bright White"=97] ("Color")
                n182 = Unbundle By Name(w366) -> ("Color Scheme"=w365:T3)
                n183 = call "Select Color.vi"("Color"=w364, "Color Scheme"=w365) -> ("Color Value"=w362:u32)  [unwired: 9 in]
                n184 = Bundle By Name(cluster=w363, "Attributes.BG"=w362) -> (w361:T5)
              }
              frame "44" {
                w370 = T4 34 items=["Black"=30, "Red"=31, "Green"=32, "Yellow"=33, "Blue"=34, "Magenta"=35, "Cyan"=36, "White"=37, "Gray"=90, "Bright Red"=91, "Bright Green"=92, "Bright Yellow"=93, "Bright Blue"=94, "Bright Magenta"=95, "Bright Cyan"=96, "Bright White"=97] ("Color")
                n185 = Unbundle By Name(w372) -> ("Color Scheme"=w371:T3)
                n186 = call "Select Color.vi"("Color"=w370, "Color Scheme"=w371) -> ("Color Value"=w368:u32)  [unwired: 9 in]
                n187 = Bundle By Name(cluster=w369, "Attributes.BG"=w368) -> (w367:T5)
              }
              frame "45" {
                w376 = T4 35 items=["Black"=30, "Red"=31, "Green"=32, "Yellow"=33, "Blue"=34, "Magenta"=35, "Cyan"=36, "White"=37, "Gray"=90, "Bright Red"=91, "Bright Green"=92, "Bright Yellow"=93, "Bright Blue"=94, "Bright Magenta"=95, "Bright Cyan"=96, "Bright White"=97] ("Color")
                n188 = Unbundle By Name(w378) -> ("Color Scheme"=w377:T3)
                n189 = call "Select Color.vi"("Color"=w376, "Color Scheme"=w377) -> ("Color Value"=w374:u32)  [unwired: 9 in]
                n190 = Bundle By Name(cluster=w375, "Attributes.BG"=w374) -> (w373:T5)
              }
              frame "46" {
                w382 = T4 36 items=["Black"=30, "Red"=31, "Green"=32, "Yellow"=33, "Blue"=34, "Magenta"=35, "Cyan"=36, "White"=37, "Gray"=90, "Bright Red"=91, "Bright Green"=92, "Bright Yellow"=93, "Bright Blue"=94, "Bright Magenta"=95, "Bright Cyan"=96, "Bright White"=97] ("Color")
                n191 = Unbundle By Name(w384) -> ("Color Scheme"=w383:T3)
                n192 = call "Select Color.vi"("Color"=w382, "Color Scheme"=w383) -> ("Color Value"=w380:u32)  [unwired: 9 in]
                n193 = Bundle By Name(cluster=w381, "Attributes.BG"=w380) -> (w379:T5)
              }
              frame "47" {
                w388 = T4 37 items=["Black"=30, "Red"=31, "Green"=32, "Yellow"=33, "Blue"=34, "Magenta"=35, "Cyan"=36, "White"=37, "Gray"=90, "Bright Red"=91, "Bright Green"=92, "Bright Yellow"=93, "Bright Blue"=94, "Bright Magenta"=95, "Bright Cyan"=96, "Bright White"=97] ("Color")
                n194 = Unbundle By Name(w390) -> ("Color Scheme"=w389:T3)
                n195 = call "Select Color.vi"("Color"=w388, "Color Scheme"=w389) -> ("Color Value"=w386:u32)  [unwired: 9 in]
                n196 = Bundle By Name(cluster=w387, "Attributes.BG"=w386) -> (w385:T5)
              }
              frame "49" {
                n197 = Unbundle By Name(w396) -> ("Color Scheme"=w395:T3, "Default BG"=w391:T4)
                n198 = call "Select Color.vi"("Color"=w391, "Color Scheme"=w395) -> ("Color Value"=w393:u32)  [unwired: 9 in]
                n199 = Bundle By Name(cluster=w394, "Attributes.BG"=w393) -> (w392:T5)
              }
              frame "90" {
                w400 = T4 90 items=["Black"=30, "Red"=31, "Green"=32, "Yellow"=33, "Blue"=34, "Magenta"=35, "Cyan"=36, "White"=37, "Gray"=90, "Bright Red"=91, "Bright Green"=92, "Bright Yellow"=93, "Bright Blue"=94, "Bright Magenta"=95, "Bright Cyan"=96, "Bright White"=97] ("Color")
                n200 = Unbundle By Name(w402) -> ("Color Scheme"=w401:T3)
                n201 = call "Select Color.vi"("Color"=w400, "Color Scheme"=w401) -> ("Color Value"=w398:u32)  [unwired: 9 in]
                n202 = Bundle By Name(cluster=w399, "Attributes.FG"=w398) -> (w397:T5)
              }
              frame "91" {
                w406 = T4 91 items=["Black"=30, "Red"=31, "Green"=32, "Yellow"=33, "Blue"=34, "Magenta"=35, "Cyan"=36, "White"=37, "Gray"=90, "Bright Red"=91, "Bright Green"=92, "Bright Yellow"=93, "Bright Blue"=94, "Bright Magenta"=95, "Bright Cyan"=96, "Bright White"=97] ("Color")
                n203 = Unbundle By Name(w408) -> ("Color Scheme"=w407:T3)
                n204 = call "Select Color.vi"("Color"=w406, "Color Scheme"=w407) -> ("Color Value"=w404:u32)  [unwired: 9 in]
                n205 = Bundle By Name(cluster=w405, "Attributes.FG"=w404) -> (w403:T5)
              }
              frame "92" {
                w412 = T4 92 items=["Black"=30, "Red"=31, "Green"=32, "Yellow"=33, "Blue"=34, "Magenta"=35, "Cyan"=36, "White"=37, "Gray"=90, "Bright Red"=91, "Bright Green"=92, "Bright Yellow"=93, "Bright Blue"=94, "Bright Magenta"=95, "Bright Cyan"=96, "Bright White"=97] ("Color")
                n206 = Unbundle By Name(w414) -> ("Color Scheme"=w413:T3)
                n207 = call "Select Color.vi"("Color"=w412, "Color Scheme"=w413) -> ("Color Value"=w410:u32)  [unwired: 9 in]
                n208 = Bundle By Name(cluster=w411, "Attributes.FG"=w410) -> (w409:T5)
              }
              frame "93" {
                w418 = T4 93 items=["Black"=30, "Red"=31, "Green"=32, "Yellow"=33, "Blue"=34, "Magenta"=35, "Cyan"=36, "White"=37, "Gray"=90, "Bright Red"=91, "Bright Green"=92, "Bright Yellow"=93, "Bright Blue"=94, "Bright Magenta"=95, "Bright Cyan"=96, "Bright White"=97] ("Color")
                n209 = Unbundle By Name(w420) -> ("Color Scheme"=w419:T3)
                n210 = call "Select Color.vi"("Color"=w418, "Color Scheme"=w419) -> ("Color Value"=w416:u32)  [unwired: 9 in]
                n211 = Bundle By Name(cluster=w417, "Attributes.FG"=w416) -> (w415:T5)
              }
              frame "94" {
                w424 = T4 94 items=["Black"=30, "Red"=31, "Green"=32, "Yellow"=33, "Blue"=34, "Magenta"=35, "Cyan"=36, "White"=37, "Gray"=90, "Bright Red"=91, "Bright Green"=92, "Bright Yellow"=93, "Bright Blue"=94, "Bright Magenta"=95, "Bright Cyan"=96, "Bright White"=97] ("Color")
                n212 = Unbundle By Name(w426) -> ("Color Scheme"=w425:T3)
                n213 = call "Select Color.vi"("Color"=w424, "Color Scheme"=w425) -> ("Color Value"=w422:u32)  [unwired: 9 in]
                n214 = Bundle By Name(cluster=w423, "Attributes.FG"=w422) -> (w421:T5)
              }
              frame "95" {
                w430 = T4 95 items=["Black"=30, "Red"=31, "Green"=32, "Yellow"=33, "Blue"=34, "Magenta"=35, "Cyan"=36, "White"=37, "Gray"=90, "Bright Red"=91, "Bright Green"=92, "Bright Yellow"=93, "Bright Blue"=94, "Bright Magenta"=95, "Bright Cyan"=96, "Bright White"=97] ("Color")
                n215 = Unbundle By Name(w432) -> ("Color Scheme"=w431:T3)
                n216 = call "Select Color.vi"("Color"=w430, "Color Scheme"=w431) -> ("Color Value"=w428:u32)  [unwired: 9 in]
                n217 = Bundle By Name(cluster=w429, "Attributes.FG"=w428) -> (w427:T5)
              }
              frame "96" {
                w436 = T4 96 items=["Black"=30, "Red"=31, "Green"=32, "Yellow"=33, "Blue"=34, "Magenta"=35, "Cyan"=36, "White"=37, "Gray"=90, "Bright Red"=91, "Bright Green"=92, "Bright Yellow"=93, "Bright Blue"=94, "Bright Magenta"=95, "Bright Cyan"=96, "Bright White"=97] ("Color")
                n218 = Unbundle By Name(w438) -> ("Color Scheme"=w437:T3)
                n219 = call "Select Color.vi"("Color"=w436, "Color Scheme"=w437) -> ("Color Value"=w434:u32)  [unwired: 9 in]
                n220 = Bundle By Name(cluster=w435, "Attributes.FG"=w434) -> (w433:T5)
              }
              frame "97" {
                w442 = T4 97 items=["Black"=30, "Red"=31, "Green"=32, "Yellow"=33, "Blue"=34, "Magenta"=35, "Cyan"=36, "White"=37, "Gray"=90, "Bright Red"=91, "Bright Green"=92, "Bright Yellow"=93, "Bright Blue"=94, "Bright Magenta"=95, "Bright Cyan"=96, "Bright White"=97] ("Color")
                n221 = Unbundle By Name(w444) -> ("Color Scheme"=w443:T3)
                n222 = call "Select Color.vi"("Color"=w442, "Color Scheme"=w443) -> ("Color Value"=w440:u32)  [unwired: 9 in]
                n223 = Bundle By Name(cluster=w441, "Attributes.FG"=w440) -> (w439:T5)
              }
              frame "100" {
                w448 = T4 90 items=["Black"=30, "Red"=31, "Green"=32, "Yellow"=33, "Blue"=34, "Magenta"=35, "Cyan"=36, "White"=37, "Gray"=90, "Bright Red"=91, "Bright Green"=92, "Bright Yellow"=93, "Bright Blue"=94, "Bright Magenta"=95, "Bright Cyan"=96, "Bright White"=97] ("Color")
                n224 = Unbundle By Name(w450) -> ("Color Scheme"=w449:T3)
                n225 = call "Select Color.vi"("Color"=w448, "Color Scheme"=w449) -> ("Color Value"=w446:u32)  [unwired: 9 in]
                n226 = Bundle By Name(cluster=w447, "Attributes.BG"=w446) -> (w445:T5)
              }
              frame "101" {
                w454 = T4 91 items=["Black"=30, "Red"=31, "Green"=32, "Yellow"=33, "Blue"=34, "Magenta"=35, "Cyan"=36, "White"=37, "Gray"=90, "Bright Red"=91, "Bright Green"=92, "Bright Yellow"=93, "Bright Blue"=94, "Bright Magenta"=95, "Bright Cyan"=96, "Bright White"=97] ("Color")
                n227 = Unbundle By Name(w456) -> ("Color Scheme"=w455:T3)
                n228 = call "Select Color.vi"("Color"=w454, "Color Scheme"=w455) -> ("Color Value"=w452:u32)  [unwired: 9 in]
                n229 = Bundle By Name(cluster=w453, "Attributes.BG"=w452) -> (w451:T5)
              }
              frame "102" {
                w460 = T4 92 items=["Black"=30, "Red"=31, "Green"=32, "Yellow"=33, "Blue"=34, "Magenta"=35, "Cyan"=36, "White"=37, "Gray"=90, "Bright Red"=91, "Bright Green"=92, "Bright Yellow"=93, "Bright Blue"=94, "Bright Magenta"=95, "Bright Cyan"=96, "Bright White"=97] ("Color")
                n230 = Unbundle By Name(w462) -> ("Color Scheme"=w461:T3)
                n231 = call "Select Color.vi"("Color"=w460, "Color Scheme"=w461) -> ("Color Value"=w458:u32)  [unwired: 9 in]
                n232 = Bundle By Name(cluster=w459, "Attributes.BG"=w458) -> (w457:T5)
              }
              frame "103" {
                w466 = T4 93 items=["Black"=30, "Red"=31, "Green"=32, "Yellow"=33, "Blue"=34, "Magenta"=35, "Cyan"=36, "White"=37, "Gray"=90, "Bright Red"=91, "Bright Green"=92, "Bright Yellow"=93, "Bright Blue"=94, "Bright Magenta"=95, "Bright Cyan"=96, "Bright White"=97] ("Color")
                n233 = Unbundle By Name(w468) -> ("Color Scheme"=w467:T3)
                n234 = call "Select Color.vi"("Color"=w466, "Color Scheme"=w467) -> ("Color Value"=w464:u32)  [unwired: 9 in]
                n235 = Bundle By Name(cluster=w465, "Attributes.BG"=w464) -> (w463:T5)
              }
              frame "104" {
                w472 = T4 94 items=["Black"=30, "Red"=31, "Green"=32, "Yellow"=33, "Blue"=34, "Magenta"=35, "Cyan"=36, "White"=37, "Gray"=90, "Bright Red"=91, "Bright Green"=92, "Bright Yellow"=93, "Bright Blue"=94, "Bright Magenta"=95, "Bright Cyan"=96, "Bright White"=97] ("Color")
                n236 = Unbundle By Name(w474) -> ("Color Scheme"=w473:T3)
                n237 = call "Select Color.vi"("Color"=w472, "Color Scheme"=w473) -> ("Color Value"=w470:u32)  [unwired: 9 in]
                n238 = Bundle By Name(cluster=w471, "Attributes.BG"=w470) -> (w469:T5)
              }
              frame "105" {
                w478 = T4 95 items=["Black"=30, "Red"=31, "Green"=32, "Yellow"=33, "Blue"=34, "Magenta"=35, "Cyan"=36, "White"=37, "Gray"=90, "Bright Red"=91, "Bright Green"=92, "Bright Yellow"=93, "Bright Blue"=94, "Bright Magenta"=95, "Bright Cyan"=96, "Bright White"=97] ("Color")
                n239 = Unbundle By Name(w480) -> ("Color Scheme"=w479:T3)
                n240 = call "Select Color.vi"("Color"=w478, "Color Scheme"=w479) -> ("Color Value"=w476:u32)  [unwired: 9 in]
                n241 = Bundle By Name(cluster=w477, "Attributes.BG"=w476) -> (w475:T5)
              }
              frame "106" {
                w484 = T4 96 items=["Black"=30, "Red"=31, "Green"=32, "Yellow"=33, "Blue"=34, "Magenta"=35, "Cyan"=36, "White"=37, "Gray"=90, "Bright Red"=91, "Bright Green"=92, "Bright Yellow"=93, "Bright Blue"=94, "Bright Magenta"=95, "Bright Cyan"=96, "Bright White"=97] ("Color")
                n242 = Unbundle By Name(w486) -> ("Color Scheme"=w485:T3)
                n243 = call "Select Color.vi"("Color"=w484, "Color Scheme"=w485) -> ("Color Value"=w482:u32)  [unwired: 9 in]
                n244 = Bundle By Name(cluster=w483, "Attributes.BG"=w482) -> (w481:T5)
              }
              frame "107" {
                w490 = T4 97 items=["Black"=30, "Red"=31, "Green"=32, "Yellow"=33, "Blue"=34, "Magenta"=35, "Cyan"=36, "White"=37, "Gray"=90, "Bright Red"=91, "Bright Green"=92, "Bright Yellow"=93, "Bright Blue"=94, "Bright Magenta"=95, "Bright Cyan"=96, "Bright White"=97] ("Color")
                n245 = Unbundle By Name(w492) -> ("Color Scheme"=w491:T3)
                n246 = call "Select Color.vi"("Color"=w490, "Color Scheme"=w491) -> ("Color Value"=w488:u32)  [unwired: 9 in]
                n247 = Bundle By Name(cluster=w489, "Attributes.BG"=w488) -> (w487:T5)
              }
            }
          }
        }
      }
    }
  }
  n248 = Bundle By Name(cluster=w6, "Buffer State.Sequence"="" ("Sequence"), "Buffer State.ESC"=FALSE ("ESC")) -> (→"Parse State":T5)
